vi "Main.vi"() -> ()   [LabVIEW 2019]
doc: "The myRIO Project template acquires acceleration data from the onboard accelerometer and displays the changes of acceleration values in a waveform chart."
uses:
  Program Files (x86)/National Instruments/LabVIEW 2019/examples/Instrument IO/Serial/support/Serial - Settings.ctl
  <vilib>/Utility/error.llb/DialogType.ctl
  <vilib>/myRIO/Instrument Drivers/Onboard IO/UART/typedef/VISA Configuration.ctl
  <vilib>/Instr/_visa.llb/VISA Flush IO Buffer Mask.ctl
  <vilib>/myRIO/Instrument Drivers/Onboard IO/DIO/typedefs/DIO Reference.ctl
  <vilib>/myRIO/Common/Instrument Driver Framework/Utilities/typedefs/myRIO Generic Hardware Reference.ctl
  <vilib>/myRIO/Common/Instrument Driver Framework/Utilities/typedefs/Hardware Version Enum.ctl
  <vilib>/myRIO/Common/Instrument Driver Framework/Utilities/typedefs/myRIO v1.0 Reference.ctl
  <vilib>/myRIO/Common/Instrument Driver Framework/Utilities/typedefs/Generic FPGA Reference.ctl
  <vilib>/myRIO/Common/Instrument Driver Framework/myRIO v1.0/DIO/typedefs/DIO Channels List.ctl
  <vilib>/myRIO/Common/Instrument Driver Framework/myRIO v1.0/DIO/typedefs/DIO Channels Enum.ctl
  <vilib>/userDefined/High Color/nirio_resource_hc.ctl
  <vilib>/myRIO/Instrument Drivers/Onboard IO/AO/typedefs/AO Reference.ctl
  <vilib>/myRIO/Common/Instrument Driver Framework/myRIO v1.0/AO/typedefs/AO Channels List.ctl
  <vilib>/myRIO/Common/Instrument Driver Framework/myRIO v1.0/AO/typedefs/AO Channels Enum.ctl
  <vilib>/myRIO/Common/Instrument Driver Framework/Utilities/typedefs/Analog Scaling Constants List.ctl
  <vilib>/myRIO/Common/Instrument Driver Framework/Utilities/typedefs/Analog Scaling Constants.ctl
  <vilib>/myRIO/Common/Instrument Driver Framework/Utilities/vis/Is FPGA Ref Available.vi
  <vilib>/myRIO/Common/Instrument Driver Framework/myRIO v1.0/DIO/vis/myRIO v1.1 Open DIO.vi
  <vilib>/myRIO/Instrument Drivers/Onboard IO/DIO/vis/Read.vi
  <vilib>/myRIO/Instrument Drivers/Onboard IO/DIO/vis/Write.vi
  <vilib>/myRIO/Common/Instrument Driver Framework/myRIO v1.0/AO/vis/myRIO v1.1 Open AO.vi
  <vilib>/myRIO/Instrument Drivers/Onboard IO/AO/vis/Write.vi
  <vilib>/myRIO/Common/Instrument Driver Framework/Utilities/vis/Validate Channels.vi
  <vilib>/myRIO/Common/Instrument Driver Framework/myRIO v1.0/DIO/vis/myRIO v1.0 Reserve DIO.vi
  <vilib>/myRIO/Common/Instrument Driver Framework/myRIO v1.0/AO/vis/myRIO v1.0 Reserve AO.vi
  <vilib>/myRIO/Common/Instrument Driver Framework/myRIO v1.0/UART/vis/myRIO v1.0 Close UART.vi
  <vilib>/myRIO/Common/Instrument Driver Framework/myRIO v1.0/Resource Manager/vis/myRIO v1.0 Reserve Channel List.vi
  <vilib>/myRIO/Common/Instrument Driver Framework/myRIO v1.0/DIO/vis/myRIO v1.0 Build MUX Configuration DIO.vi
  <vilib>/myRIO/Common/Instrument Driver Framework/myRIO v1.0/AO/vis/myRIO v1.0 Build MUX Configuration AO.vi
  <vilib>/myRIO/Common/Instrument Driver Framework/myRIO v1.0/Resource Manager/vis/myRIO v1.0 Reserve Channel.vi
  <vilib>/myRIO/Common/Instrument Driver Framework/myRIO v1.0/Resource Manager/vis/myRIO v1.0 Unreserve Channel.vi
  <vilib>/myRIO/Common/Instrument Driver Framework/myRIO v1.0/Resource Manager/vis/myRIO v1.0 Create Configuration List.vi
  <vilib>/myRIO/Common/Instrument Driver Framework/myRIO v1.0/Resource Manager/vis/myRIO v1.0 Build Mutex Name.vi
  <vilib>/Instr/_visa.llb/VISA Configure Serial Port (Serial Instr).vi
  <vilib>/Instr/_visa.llb/VISA Configure Serial Port (Instr).vi
  <vilib>/Utility/VariantDataType/GetNumericInfo.vi
  <vilib>/Utility/error.llb/Error Cluster From Error Code.vi
  <vilib>/myRIO/Common/Instrument Driver Framework/myRIO v1.0/myRIO v1.1 Open.vi
  <vilib>/myRIO/Common/Instrument Driver Framework/Utilities/vis/IO Manager.vi
  <vilib>/myRIO/Common/Instrument Driver Framework/Utilities/vis/Configuration Manager.vi
  <vilib>/myRIO/Common/Instrument Driver Framework/myRIO v1.0/Resource Manager/vis/myRIO v1.0 Configure IO.vi
  <vilib>/myRIO/Common/Instrument Driver Framework/myRIO v1.0/myRIO v1.0 Close.vi
  <vilib>/myRIO/Common/Instrument Driver Framework/myRIO v1.0/DIO/vis/myRIO v1.0 Write DIO.vi
  <vilib>/myRIO/Common/Instrument Driver Framework/myRIO v1.0/DIO/vis/myRIO v1.0 Read DIO.vi
  <vilib>/addons/control/pid/pid.llb/PID (DBL).vi
  <vilib>/myRIO/Common/Instrument Driver Framework/myRIO v1.0/AO/vis/myRIO v1.0 Get Scaling Constants AO.vi
  <vilib>/myRIO/Common/Instrument Driver Framework/myRIO v1.0/AO/vis/myRIO v1.0 Write AO.vi
  <vilib>/myRIO/Common/Instrument Driver Framework/Utilities/vis/FPGA Ref Manager.vi
  <vilib>/myRIO/Common/Instrument Driver Framework/myRIO v1.0/myRIO v1.0 Reset FPGA.vi
  <vilib>/myRIO/Common/Instrument Driver Framework/myRIO v1.0/IRQ/vis/myRIO v1.0 IRQ Info FGV.vi
  <vilib>/myRIO/Common/Instrument Driver Framework/myRIO v1.0/IRQ/vis/myRIO v1.0 Timer IRQ Info FGV.vi
  <vilib>/myRIO/Common/Instrument Driver Framework/myRIO v1.0/IRQ/vis/myRIO v1.0 ISR Agent.vi
  <vilib>/myRIO/Instrument Drivers/Utilities/vis/Reset Index.vi
  <vilib>/myRIO/Common/Instrument Driver Framework/myRIO v1.0/Resource Manager/vis/myRIO v1.0 Block Write Resource Manager.vi
  <vilib>/myRIO/Express VI/Onboard IO/DO/DO Express VI.xnode
  <vilib>/myRIO/Instrument Drivers/Onboard IO/DIO/vis/myRIO DIO Open.xnode
  <vilib>/myRIO/Express VI/Onboard IO/DI/DI Express VI.xnode
  <vilib>/myRIO/Express VI/Onboard IO/AO/AO Express VI.xnode
  <vilib>/myRIO/Instrument Drivers/Onboard IO/AO/vis/myRIO AO Open.xnode
  <vilib>/myRIO/Instrument Drivers/Utilities/Utilities.lvlib
  <vilib>/myRIO/Instrument Drivers/Onboard IO/UART/UART.lvlib
  <vilib>/myRIO/Instrument Drivers/Onboard IO/DIO/DIO.lvlib
  <vilib>/myRIO/Instrument Drivers/Onboard IO/AO/AO.lvlib
  <vilib>/addons/control/pid/NI_PID_pid.lvlib
  <vilib>/Analysis/NI_AALBase.lvlib
  <vilib>/ptbypt/NI_PtbyPt.lvlib
panel:
  out "?":bool
  out "?":bool
  out "Read Errors":i32
  in  "type of dialog (OK msg:1)":T1 items=["no dialog", "OK message", "continue or stop message", "OK message + warnings", "continue/stop + warnings"]
  out "encoder":dynamicdata(graph)
  out "Waveform Chart 2":dynamicdata(graph)
  out "x*y":dbl
  in  "Termination Character":u8=10 format="%.0x"
  in  "End Write on Termination Character?":bool=TRUE
  in  "End Read on Termination Character?":bool=TRUE
  in  "Write String":string="OUTPUT RS422\n"
  in  "Serial Settings":T2={"baud rate"=921600, "data bits"=8, "parity"=enum."None", "stop bits"=10, "flow control"=0} {"flow control" items=["None"=0, "XON/XOFF"=1, "RTS/CTS"=2, "DTR/DSR"=4]; "stop bits" items=["1.0"=10, "1.5"=15, "2.0"=20]; "data bits" min=5 max=8 step=1; "baud rate" items=["921600"=921600, "9600"=9600, "115200"=115200]}
  in  "Assert DTR?":bool
  in  "VISA Refnum in":refnum<visa-resource-name>="ASRL1::INSTR"
  in  "Stop":bool
  in  "Forward":bool
  in  "Reverse":bool
  out "Laser Error":bool
  in  "Slide":dbl(slide) min=0.0 max=2.5 step=0.1 scale=0.0..9.0
  in  "Laser ON":bool
  out "Load":dynamicdata(graph)
  out "Load":dbl
  out "encoder":dbl
  out "timer":dbl
  out "Serial Settings:Number of Bytes at Serial Port":u32
  out "error out 2":errorcluster
  in  "error in (no error)":errorcluster
  out "Arduino Read":string
  in  "Stop":bool
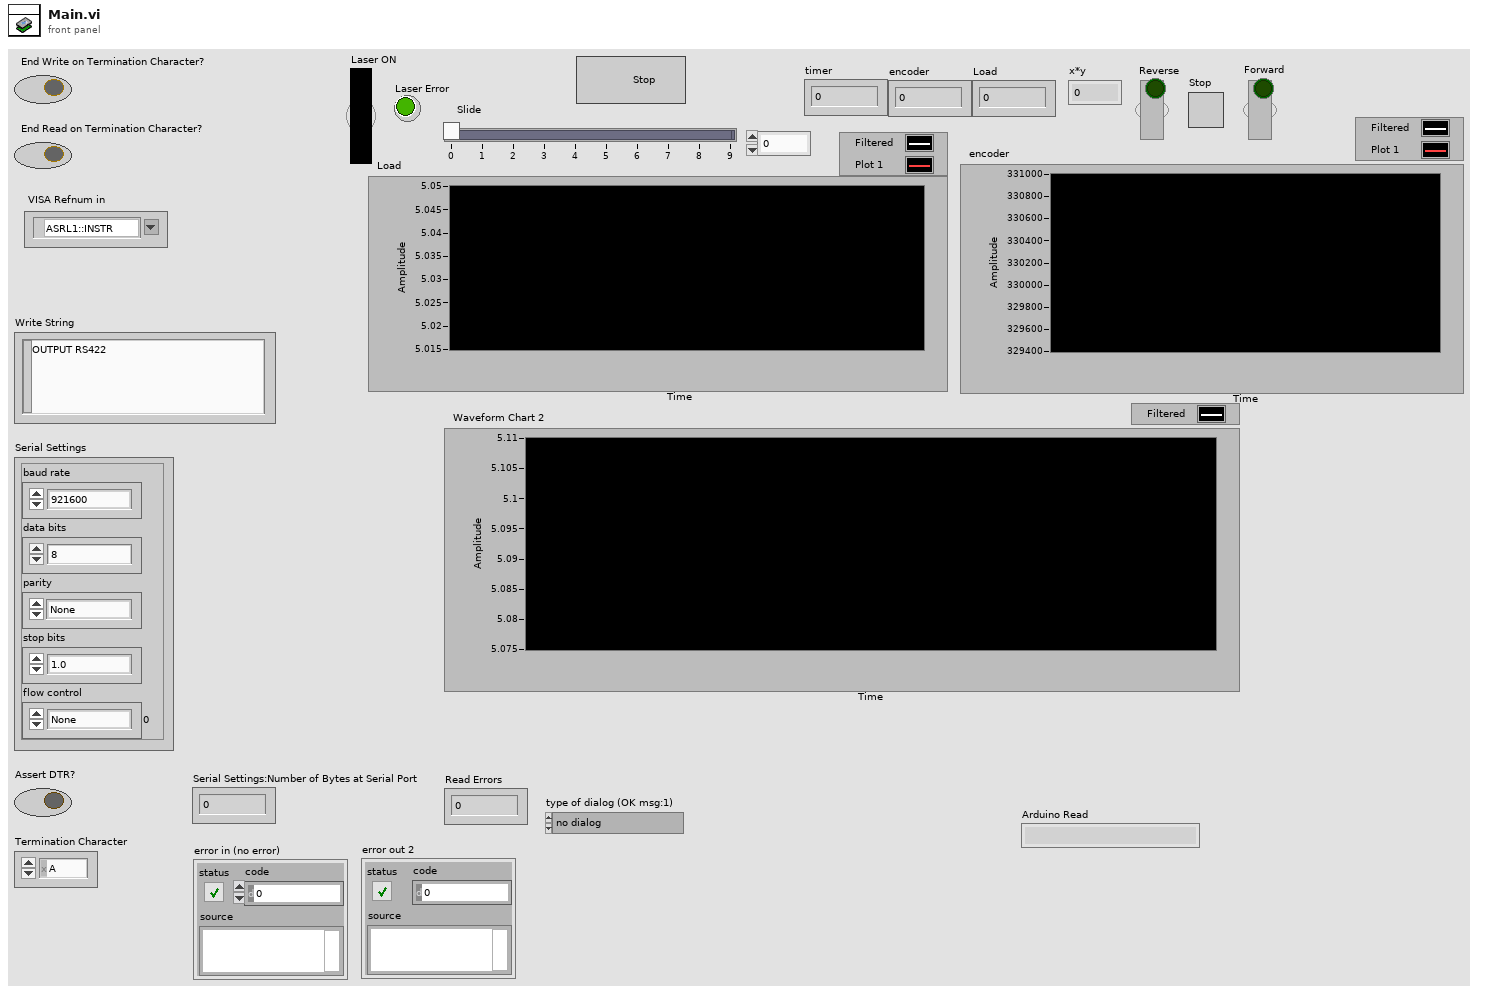
[diagram p1: front panel]
types:
  T1 = typedef "DialogType.ctl" = u16
  T2 = typedef "Serial - Settings.ctl" = cluster{"baud rate":u32, "data bits":u16, "parity":enum16{"None", "Odd", "Even", "Mark", "Space"}, "stop bits":u16, "flow control":u16}
  T3 = typedef "DIO.lvlib/DIO Reference.ctl" = cluster{"myRIO Reference":T4, "DIO Channels List":T8}
  T4 = typedef "myRIO Generic Hardware Reference.ctl" = cluster{"myRIO Model":T5, "myRIO Hardware Reference":T6}
  T5 = typedef "Hardware Version Enum.ctl" = enum16{"Unknown", "myRIO-1900", "myRIO-1950", "roboRIO", "NI ELVIS RIO CM", "ELVIS III"}
  T6 = typedef "myRIO v1.0 Reference.ctl" = cluster{"Generic FPGA Reference":T7, "Allow multiple opens":bool}
  T7 = typedef "Generic FPGA Reference.ctl" = refnum<k20>
  T8 = typedef "DIO Channels List.ctl" = T9[]
  T9 = typedef "DIO Channels Enum.ctl" = enum16{"Not Connected", "C/DIO0", "C/DIO1", "C/DIO2", "C/DIO3", "C/DIO4", "C/DIO5", "C/DIO6", "C/DIO7", "A/DIO0", "A/DIO1", "A/DIO2", "A/DIO3", "A/DIO4", "A/DIO5", "A/DIO6", "A/DIO7", "A/DIO8", "A/DIO9", "A/DIO10", "A/DIO11", "A/DIO12", "A/DIO13", "A/DIO14", "A/DIO15", "A/DIO16", "A/DIO17", "A/DIO18", "A/DIO19", "B/DIO0", "B/DIO1", "B/DIO2", "B/DIO3", "B/DIO4", "B/DIO5", "B/DIO6", "B/DIO7", "B/DIO8", "B/DIO9", "B/DIO10", "B/DIO11", "B/DIO12", "B/DIO13", "B/DIO14", "B/DIO15", "B/DIO16", "B/DIO17", "B/DIO18", "B/DIO19", "LED0", "LED1", "LED2", "LED3", "Button0", "DIO/DIO0", "DIO/DIO1", "DIO/DIO2", "DIO/DIO3", "DIO/DIO4", "DIO/DIO5", "DIO/DIO6", "DIO/DIO7", "DIO/DIO8", "DIO/DIO9", "SPI/CS0", "SPI/CS1", "SPI/CS2", "SPI/CS3", "LED RADIO (Green)", "LED RADIO (Red)", "LED COMM (Green)", "LED COMM (Red)", "LED MODE (Green)", "LED MODE (Red)"}
  T10 = typedef "nirio_resource_hc.ctl" = tag
  T11 = cluster{"proportional gain (Kc)":dbl, "integral time (Ti, min)":dbl, "derivative time (Td, min)":dbl}
  T12 = typedef "AO.lvlib/AO Reference.ctl" = cluster{"myRIO Reference":T4, "AO Channel List":T13, "AO Scaling Constant List":T15}
  T13 = typedef "AO Channels List.ctl" = T14[]
  T14 = typedef "AO Channels Enum.ctl" = enum16{"Not Connected", "AudioOut/Left", "AudioOut/Right", "C/AO0", "C/AO1", "A/AO0", "A/AO1", "B/AO0", "B/AO1"}
  T15 = typedef "Analog Scaling Constants List.ctl" = T16[]
  T16 = typedef "Analog Scaling Constants.ctl" = cluster{"LSB Weight (Volts)":dbl, "Offset (Volts)":dbl, "Signed?":bool}
  T17 = typedef "VISA Flush IO Buffer Mask.ctl" = u16
  T18 = typedef "UART.lvlib/VISA Configuration.ctl" = cluster{"baud rate (9600)":u32, "data bits (8)":u16, "parity (0:none)":enum16{"None", "Odd", "Even", "Mark", "Space"}, "stop bits (10: 1 bit)":u16, "flow control (0:none)":u16, "termination char\n(0xA = '\\n' = LF) ":u8, "Enable Termination\nChar (T)":bool, "timeout (10sec)":u32}
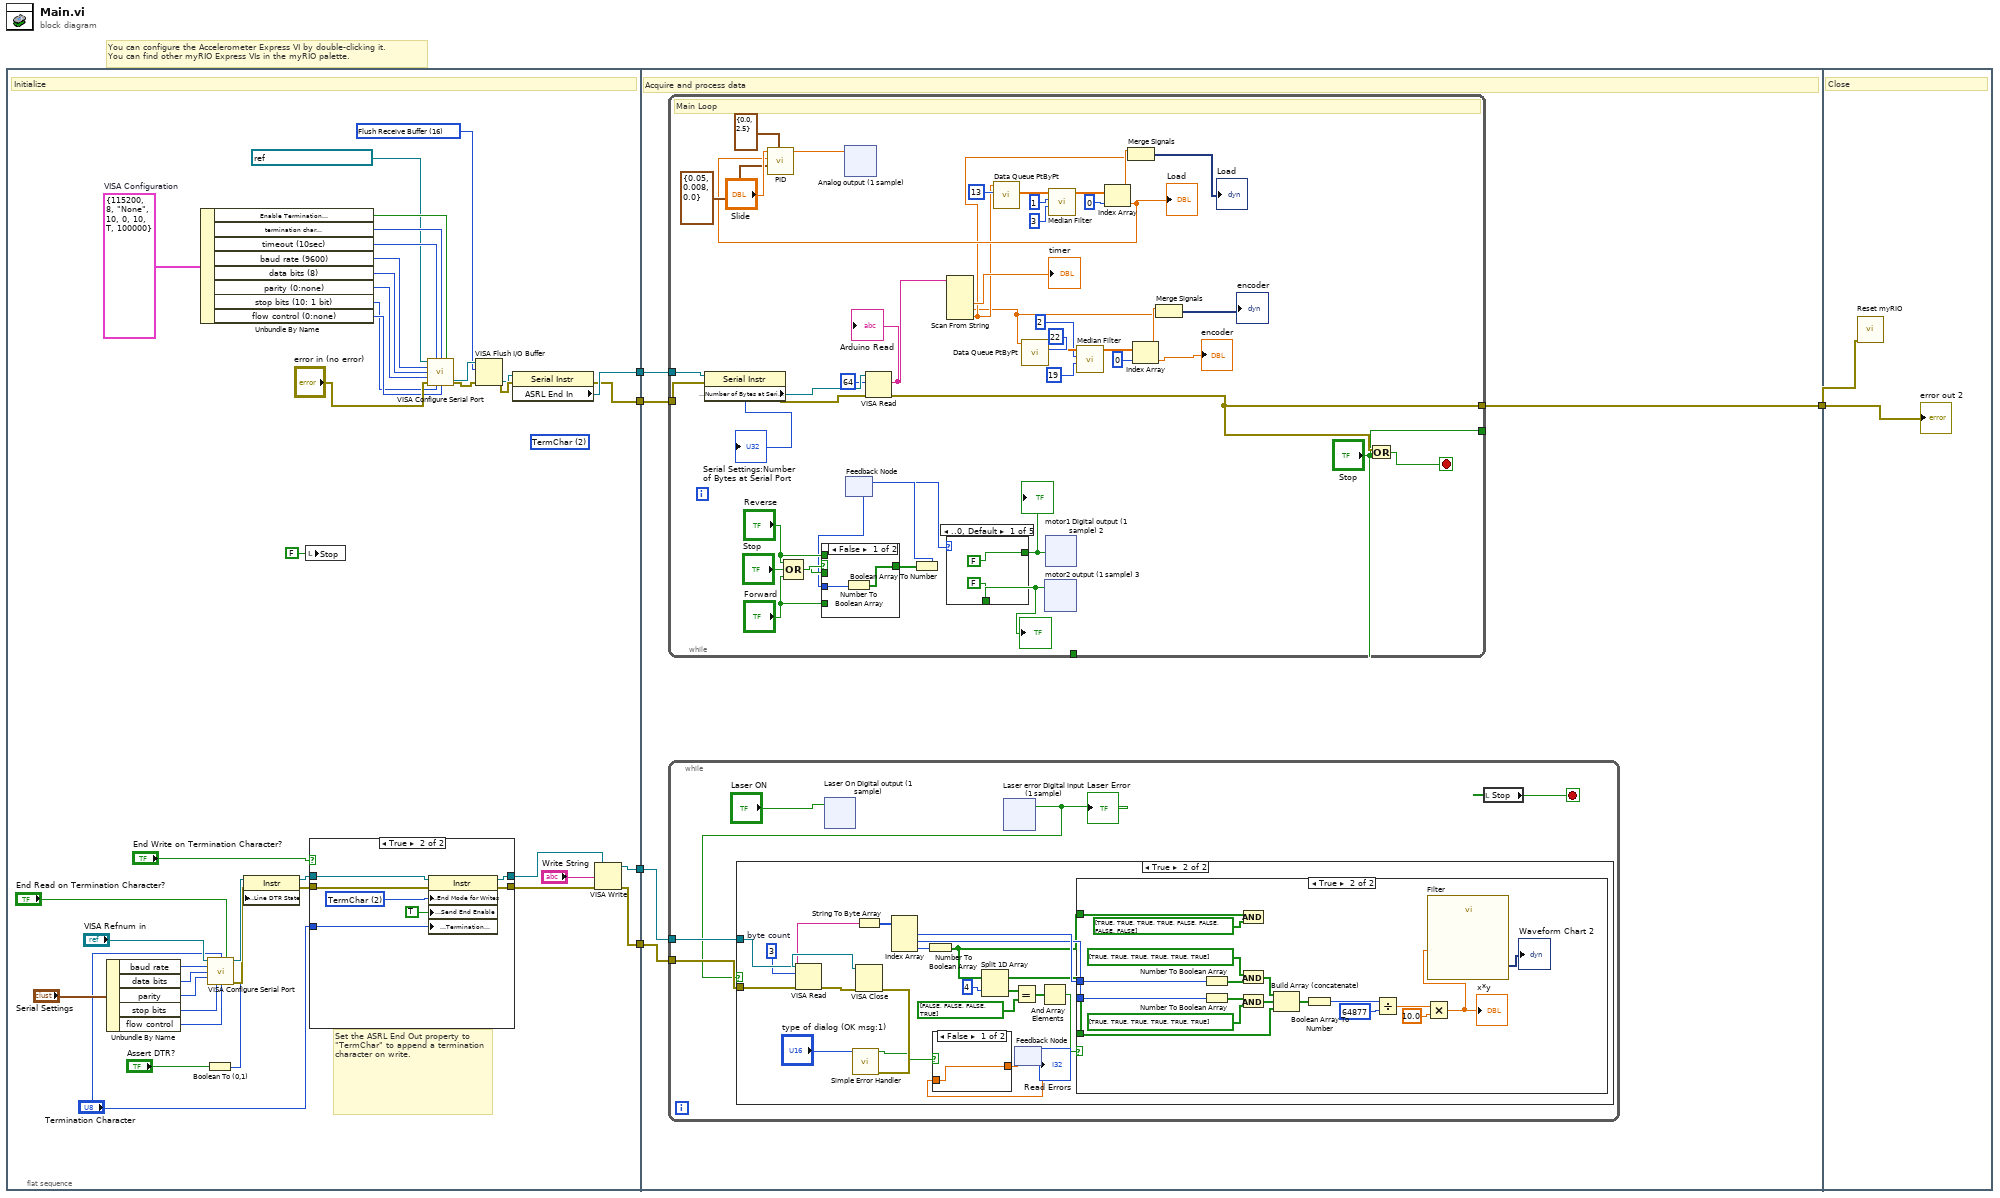
[diagram p0: block diagram]
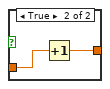
[diagram p4: hidden frame]
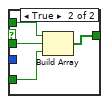
[diagram p6: hidden frame]
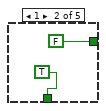
[diagram p7: hidden frame]
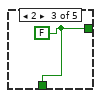
[diagram p8: hidden frame]
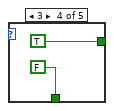
[diagram p9: hidden frame]
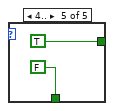
[diagram p10: hidden frame]
diagram:
  # "You can configure the Accelerometer Express VI by double-clicking it.\nYou can find other myRIO Express VIs in the myRIO palette."
  n1 = flat-sequence {
    tunnel: [w29] -> w4
    tunnel: [w28] -> w3
    tunnel: [w8] -> w2
    tunnel: [w7] -> w1
    tunnel: [w59] -> w5
    tunnel: w4 -> [w58]
    tunnel: w3 -> [w57]
    tunnel: w2 -> [w56]
    tunnel: w1 -> [w55]
    tunnel: w5 -> [w342]
    frame #0 {
      (unwired) u16 2 items=["None", "Last Bit", "TermChar"] ("Serial Settings:End Mode for Reads")
      w32 = T17 16 items=["Flush Receive Buffer"=16, "Write Transmit Buffer to Device"=32, "Flush Receive Buffer (No I/O)"=64, "Flush Transmit Buffer"=128] ("Mask")
      w31 = T18 {"baud rate (9600)"=115200, "data bits (8)"=8, "parity (0:none)"=enum."None", "stop bits (10: 1 bit)"=10, "flow control (0:none)"=0, "termination char\n(0xA = '\\n' = LF) "=10, "Enable Termination\nChar (T)"=TRUE, "timeout (10sec)"=100000}  # VISA Configuration
      # "Set the ASRL End Out property to \"TermChar\" to append a termination character on write."
      # "Initialize"
      n2 = Unbundle By Name("Serial Settings") -> ("baud rate"=w21:u32, "data bits"=w20:u16, "parity"=w19:enum16{"None", "Odd", "Even", "Mark", "Space"}, "stop bits"=w18:u16, "flow control"=w17:u16)
      n3 = Unbundle By Name(w31) -> ("Enable Termination\nChar (T)"=w39:bool, "termination char\n(0xA = '\\n' = LF)"=w41:u8, "timeout (10sec)"=w38:u32, "baud rate (9600)"=w33:u32, "data bits (8)"=w34:u16, "parity (0:none)"=w35:enum16{"None", "Odd", "Even", "Mark", "Space"}, "stop bits (10: 1 bit)"=w36:u16, "flow control (0:none)"=w37:u16)
      n4 = Boolean To (0,1)(Boolean="Assert DTR?") -> (0, 1=w23:i16)
      n5 = call-poly "VISA Configure Serial Port"("VISA resource name"="VISA Refnum in", "termination char\n(0xA = '\\n' = LF)"="Termination Character", "Enable Termination\nChar (T)"="End Read on Termination Character?", "baud rate (921600)"=w21, "data bits (8)"=w20, "parity (0:none)"=w19, "stop bits (10: 1 bit)"=w18, "flow control (0:none)"=w17) -> ("VISA resource name out"=w26:refnum<visa-resource-name>, "error out"=w25:errorcluster)  [unwired: 2 in, 4 out]
      n6 = property class="Instr"(reference=w26, error in=w25, "Serial Settings:Modem Line Settings:Line DTR State"=w23) -> (reference out=w12:refnum<visa-resource-name>, error out=w13:errorcluster)
      n7 = local write "Stop"(FALSE ("Stop")) -> ()
      n8 = case shown="True" "End Write on Termination Character?" {
        tunnel: w12 -> [w46 w54]
        tunnel: w13 -> [w47 w53]
        tunnel: [w46 w52] -> w11
        tunnel: [w47 w51] -> w14
        tunnel: "Termination Character" -> [_ w49]
        frame False {
        }
        frame True {
          w50 = u16 2 items=["None", "LastBit", "TermChar", "Break"] ("Serial Settings:Serial End Mode for Writes")
          n9 = property class="Instr"(reference=w54, error in=w53, "Serial Settings:End Mode for Writes"=w50, "Message Based Settings:Send End Enable"=TRUE, "Message Based Settings:Termination Character"=w49) -> (reference out=w52:refnum<visa-resource-name>, error out=w51:errorcluster)
        }
      }
      n10 = call-poly "VISA Configure Serial Port"("VISA resource name"=refnum<visa-resource-name> "ASRL2::INSTR", "timeout (10sec)"=w38, "termination char\n(0xA = '\\n' = LF)"=w41, "Enable Termination\nChar (T)"=w39, "baud rate (9600)"=w33, "data bits (8)"=w34, "parity (0:none)"=w35, "error in (no error)"="error in (no error)", "stop bits (10: 1 bit)"=w36, "flow control (0:none)"=w37) -> ("VISA resource name out"=w43:refnum<visa-resource-name>, "error out"=w42:errorcluster)  [unwired: 4 in]
      n11 = VISA Flush I/O Buffer(VISA resource name=w43, mask (16)=w32, error in (no error)=w42) -> (VISA resource name out=w44:refnum<visa-resource-name>, error out=w45:errorcluster)
      n12 = property class="Serial Instr" props=["ASRL End In"](reference=w44, error in=w45) -> (reference out=w29:refnum<visa-resource-name>, error out=w28:errorcluster)  [unwired: 1 out]
      n13 = VISA Write(VISA resource name=w11, write buffer="Write String", error in (no error)=w14) -> (VISA resource name out=w7:refnum<visa-resource-name>, error out=w8:errorcluster)  [unwired: 1 out]
    }
    frame #1 {
      # "Acquire and process data"
      n14 = while {
        tunnel: [w216] -> w59
        tunnel: w58 -> [w215]
        tunnel: w57 -> [w214]
        tunnel: ["Stop"] -> _
        tunnel: ["Stop"] -> _
        stop <- w219 stop-if-true
        # "Main Loop"
        n15 = property class="Serial Instr"(reference=w215, error in=w214) -> (reference out=w218:refnum<visa-resource-name>, error out=w210:errorcluster, "Serial Settings:Number of Bytes at Serial Port"=→"Serial Settings:Number of Bytes at Serial Port":u32)
        n16 = Compound Arithmetic op=OR("Reverse", "Stop", "Forward") -> (w205:bool)
        n17 = feedback #1() -> (w199:u32)  [unwired: 1 in]
        n18 = case shown="False" w205 {
          tunnel: "Forward" -> [_ w225]
          tunnel: "Stop" -> [_ w224]
          tunnel: "Reverse" -> [_ w223]
          tunnel: [w220 w222] -> w201
          tunnel: w199 -> [w221 _]
          frame False {
            n19 = Number To Boolean Array(number=w221) -> (Boolean array=w220:bool[])
          }
          frame True {
            n20 = Build Array(w223, w224, w225) -> (w222:bool[])
          }
        }
        n21 = VISA Read(VISA resource name=w218, byte count=u32 64, error in (no error)=w210) -> (read buffer=w212:string, error out=w216:errorcluster)  [unwired: 2 out]
        "Arduino Read" <- w212
        n22 = Boolean Array To Number(Boolean array=w201) -> (number=w200:u32)
        n23 = feedback-in #1(w200) -> ()
        n24 = case shown="..0, Default" w199 {
          tunnel: [FALSE FALSE w230 TRUE TRUE] -> w178
          tunnel: [FALSE TRUE w230 FALSE FALSE] -> w179
          frame ..0, Default {
          }
          frame 1 {
          }
          frame 2 {
            w230 = FALSE
          }
          frame 3 {
          }
          frame 4.. {
          }
        }
        "?" <- w179
        "?" <- w178
        n25 = Scan From String(input string=w212) -> (output 1=→"timer":dbl, output 2=w180:dbl, output 3=w192:dbl)  [unwired: 6 in, 3 out]
        n26 = call <vilib>:"Data Queue PtByPt.vi"("sample length"=13, "input data point"=w192) -> ("Current Queue"=w197:dbl[])  [unwired: 5 in, 4 out]
        n27 = call <vilib>:"Data Queue PtByPt.vi"("sample length"=22, "input data point"=w180) -> ("Current Queue"=w187:dbl[])  [unwired: 5 in, 4 out]
        n28 = xnode "motor2 output (1 sample) 3"("C/DIO3 (DIO3)"=w179) -> ()  [unwired: 1 in, 1 out]
        n29 = xnode "motor1 Digital output (1 sample) 2"("C/DIO2 (DIO2)"=w178) -> ()  [unwired: 1 in, 1 out]
        n30 = call <vilib>:"Median Filter.vi"("right rank"=3, "left rank"=1, "X"=w197) -> ("Filtered X"=w196:dbl[])  [unwired: 7 in, 1 out]
        n31 = call <vilib>:"Median Filter.vi"("right rank"=19, "left rank"=2, "X"=w187) -> ("Filtered X"=w186:dbl[])  [unwired: 7 in, 1 out]
        n32 = Index Array(array=w196, index=0) -> (element=w194:dbl)
        "Load" <- w194
        n33 = call-poly <vilib>:"PID.vi"("output range"=cluster{"output high":dbl, "output low":dbl} {"output high"=0.0, "output low"=2.5}, "PID gains"=T11 {"proportional gain (Kc)"=0.05, "integral time (Ti, min)"=0.008, "derivative time (Td, min)"=0.0}, "process variable"=w194, "setpoint"="Slide") -> ("output"=w209:dbl)  [unwired: 6 in, 1 out]
        n34 = xnode "Analog output (1 sample)"("C/AO0 (AO0)"=w209) -> ()  [unwired: 1 in, 1 out]
        n35 = Merge Signals(w194, w192) -> (→"Load":dynamicdata)
        n36 = Index Array(array=w186, index=0) -> (element=w181:dbl)
        "encoder" <- w181
        n37 = Merge Signals(w181, w180) -> (→"encoder":dynamicdata)
        n38 = Or(x=w216, y="Stop") -> (x .or. y?=w219:bool)
      }
      n39 = while {
        tunnel: w56 -> [w64]
        tunnel: w55 -> [w63]
        stop <- w62 stop-if-true
        n40 = xnode "Laser On Digital output (1 sample)"("C/DIO0 (DIO0)"="Laser ON") -> ()  [unwired: 1 in, 1 out]
        n41 = xnode "Laser error Digital input (1 sample)"() -> ("C/DIO1 (DIO1)"=w60:bool)  [unwired: 1 in, 1 out]
        "Laser Error" <- w60
        n42 = case shown="True" w60 {
          tunnel: w64 -> [_ w72]
          tunnel: w63 -> [_ w71]
          frame False {
          }
          frame True {
            w70 = u32 3  # byte count
            n43 = VISA Read(VISA resource name=w71, byte count=w70, error in (no error)=w72) -> (VISA resource name out=w85:refnum<visa-resource-name>, read buffer=w67:string, error out=w86:errorcluster)  [unwired: 1 out]
            n44 = String To Byte Array(string=w67) -> (unsigned byte array=w83:u8[])
            n45 = VISA Close(VISA resource name=w85, error in (no error)=w86) -> (error out=w84:errorcluster)
            n46 = call <vilib>:"Simple Error Handler.vi"("type of dialog (OK msg:1)"="type of dialog (OK msg:1)", "error in (no error)"=w84) -> ("error?"=w68:bool)  [unwired: 7 out]
            n47 = Index Array(array=w83) -> (element #1=w82:u8, element #2=w81:u8, element #3=w80:u8)  [unwired: 3 in]
            n48 = Number To Boolean Array(number=w80) -> (Boolean array=w79:bool[])
            n49 = Split 1D Array(array=w79, index=4) -> (first subarray=w73:bool[], second subarray=w74:bool[])
            n50 = Equal?(x=w74, y=bool[] [FALSE, FALSE, FALSE, TRUE]) -> (x = y?=w75:bool[])
            n51 = feedback #2() -> (w65:dbl)  [unwired: 1 in]
            "Read Errors" <- w65
            n52 = case shown="False" w68 {
              tunnel: w65 -> [w87 w89]
              tunnel: [w87 w88] -> w66
              frame False {
              }
              frame True {
                n53 = Increment(x=w89) -> (x+1=w88:dbl)
              }
            }
            n54 = feedback-in #2(w66) -> ()
            n55 = And Array Elements(Boolean array=w75) -> (logical AND=w76:bool)
            n56 = case shown="True" w76 {
              tunnel: w82 -> [_ w107]
              tunnel: w81 -> [_ w105]
              tunnel: w79 -> [_ w93]
              tunnel: w73 -> [_ w92]
              frame False {
              }
              frame True {
                n57 = Number To Boolean Array(number=w107) -> (Boolean array=w94:bool[])
                n58 = Number To Boolean Array(number=w105) -> (Boolean array=w104:bool[])
                n59 = And(x=w93, y=bool[] [TRUE, TRUE, TRUE, TRUE, FALSE, FALSE, FALSE, FALSE] ("x")) -> ()  [unwired: 1 out]
                n60 = And(x=bool[] [TRUE, TRUE, TRUE, TRUE, TRUE, TRUE], y=w94) -> (x .and. y?=w95:bool[])
                n61 = And(x=w104, y=bool[] [TRUE, TRUE, TRUE, TRUE, TRUE, TRUE] ("x")) -> (x .and. y?=w96:bool[])
                n62 = Build Array (concatenate)(w95, w96, w92) -> (w101:bool[])
                n63 = Boolean Array To Number(Boolean array=w101) -> (number=w100:u32)
                n64 = Divide(x=w100, y=u32 64877) -> (x/y=w98:dbl)
                n65 = Multiply(x=w98, y=10.0) -> (x*y=w91:dbl)
                "x*y" <- w91
                n66 = call "Filter"("Signal"=w91) -> ("Filtered Signal"=→"Waveform Chart 2":dynamicdata)  [unwired: 9 in, 1 out]
              }
            }
          }
        }
        n67 = local read "Stop"() -> (w62:bool)
      }
    }
    frame #2 {
      # "Close"
      n68 = call <vilib>:"Reset myRIO.vi"("error in (no error)"=w342) -> ()  [unwired: 10 in, 1 out]
      "error out 2" <- w342
    }
  }
